vi "FlexRay_FR_Tab.vi"(7 "Fold Data":bool, 8 "error in (no error)":errorcluster, 9 "FR_Buffer":T1[](array[typedef]), 10 "FlexRay_Data IN":T2={"Communication message"={"Sender"="", "receiver"="", "message"="", "data"=variant}, "error in"={"status"=FALSE, "code"=0, "source"=""}, "Data"={"FR_Frame_Buffer"=[], "Config"={"DLL_PATH"=path "", "Project_PATH"=path "", "BLF_Log_PATH"=path "", "Read message type"=1, "Channel"=0, "REC_Channel"=0, "ChannelMask"=0, "ActualPayloadLength"=0, "CycleNumber"=0, "SlotId"=0, "Send_Array"=[1, 2, 3, 4, 5, 6, 7, 8, 9, 10, 11]}, "AsynCall?"=FALSE, "XML_Data"={"XML Path"=path "", "XML loading channel"=0}, "DataBase_array"=refnum}} {"Data"."XML_Data"."XML loading channel" items=["CHN1", "CHN2", "CHN3", "CHN4", "CHN5", "CHN6", "CHN7", "CHN8", "CHN9", "CHN10", "CHN11", "CHN12", "CHN13", "CHN14", "CHN15", "CHN16", "CHN17", "CHN18", "CHN19", "CHN20", "CHN21", "CHN22", "CHN23", "CHN24", "CHN25", "CHN26", "CHN27", "CHN28", "CHN29", "CHN30", "CHN31", "CHN32"]; "Data"."Config"."Send_Array" format="%.0x"; "Data"."Config"."ChannelMask" items=["reserved", "A", "B", "AB"]; "Data"."Config"."REC_Channel" items=["CHN1", "CHN2", "CHN3", "CHN4", "CHN5", "CHN6", "CHN7", "CHN8", "CHN9", "CHN10", "CHN11", "CHN12", "CHN13", "CHN14", "CHN15", "CHN16", "CHN17", "CHN18", "CHN19", "CHN20", "CHN21", "CHN22", "CHN23", "CHN24", "CHN25", "CHN26", "CHN27", "CHN28", "CHN29", "CHN30", "CHN31", "CHN32"]; "Data"."Config"."Channel" items=["CHN1", "CHN2", "CHN3", "CHN4", "CHN5", "CHN6", "CHN7", "CHN8", "CHN9", "CHN10", "CHN11", "CHN12", "CHN13", "CHN14", "CHN15", "CHN16", "CHN17", "CHN18", "CHN19", "CHN20", "CHN21", "CHN22", "CHN23", "CHN24", "CHN25", "CHN26", "CHN27", "CHN28", "CHN29", "CHN30", "CHN31", "CHN32"]; "Data"."Config"."Read message type" items=["Only read received messages", "Receive&send messages"]}, 11 "MulticolumnListbox in":refnum<vi>) -> (2 "FlexRay_Data":T2={"Communication message"={"Sender"="", "receiver"="", "message"="", "data"=variant}, "error in"={"status"=FALSE, "code"=0, "source"=""}, "Data"={"FR_Frame_Buffer"=[], "Config"={"DLL_PATH"=path "", "Project_PATH"=path "", "BLF_Log_PATH"=path "", "Read message type"=1, "Channel"=0, "REC_Channel"=0, "ChannelMask"=0, "ActualPayloadLength"=0, "CycleNumber"=0, "SlotId"=0, "Send_Array"=[1, 2, 3, 4, 5, 6, 7, 8, 9, 10, 11]}, "AsynCall?"=FALSE, "XML_Data"={"XML Path"=path "", "XML loading channel"=0}, "DataBase_array"=refnum}} {"Data"."XML_Data"."XML loading channel" items=["CHN1", "CHN2", "CHN3", "CHN4", "CHN5", "CHN6", "CHN7", "CHN8", "CHN9", "CHN10", "CHN11", "CHN12", "CHN13", "CHN14", "CHN15", "CHN16", "CHN17", "CHN18", "CHN19", "CHN20", "CHN21", "CHN22", "CHN23", "CHN24", "CHN25", "CHN26", "CHN27", "CHN28", "CHN29", "CHN30", "CHN31", "CHN32"]; "Data"."Config"."Send_Array" format="%.0x"; "Data"."Config"."ChannelMask" items=["reserved", "A", "B", "AB"]; "Data"."Config"."REC_Channel" items=["CHN1", "CHN2", "CHN3", "CHN4", "CHN5", "CHN6", "CHN7", "CHN8", "CHN9", "CHN10", "CHN11", "CHN12", "CHN13", "CHN14", "CHN15", "CHN16", "CHN17", "CHN18", "CHN19", "CHN20", "CHN21", "CHN22", "CHN23", "CHN24", "CHN25", "CHN26", "CHN27", "CHN28", "CHN29", "CHN30", "CHN31", "CHN32"]; "Data"."Config"."Channel" items=["CHN1", "CHN2", "CHN3", "CHN4", "CHN5", "CHN6", "CHN7", "CHN8", "CHN9", "CHN10", "CHN11", "CHN12", "CHN13", "CHN14", "CHN15", "CHN16", "CHN17", "CHN18", "CHN19", "CHN20", "CHN21", "CHN22", "CHN23", "CHN24", "CHN25", "CHN26", "CHN27", "CHN28", "CHN29", "CHN30", "CHN31", "CHN32"]; "Data"."Config"."Read message type" items=["Only read received messages", "Receive&send messages"]})   [LabVIEW 2014]
uses:
  Typedef/TLibFLexRay.ctl
  Typedef/FlexRay_Data.ctl
  Typedef/FlexRay_Config.ctl
  DataBase/Typedef/CAN/TCANSignal.ctl
  DataBase/Typedef/LIN/TLINSignal.ctl
  DataBase/Typedef/FlexRay/TFlexRaySignal.ctl
  DataBase/Typedef/TDBSignalProperties.ctl
  DataBase/Typedef/TDBFrameProperties.ctl
  DataBase/Typedef/TDBECUProperties.ctl
  DataBase/Typedef/TDBProperties.ctl
  DataBase/Typedef/DataBase_array.ctl
  DataBase/Typedef/DataBase_array_index.ctl
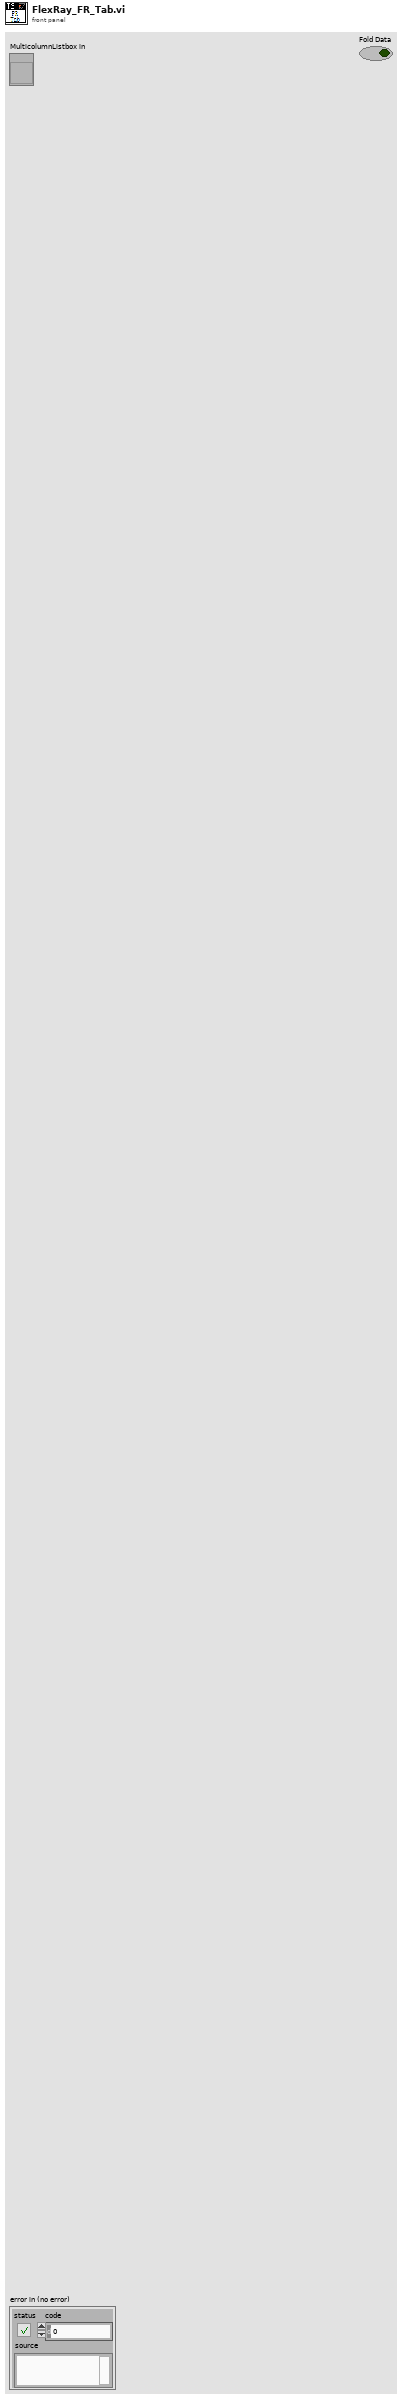
[diagram p1: front panel]
types:
  T1 = typedef "TLibFLexRay.ctl" = cluster{"FIdxChn":u8, "FChannelMask":u8, "FDir":u8, "FPayloadLength":u8, "FActualPayloadLength":u8, "FCycleNumber":u8, "FCCType":u8, "FFrameType":u8, "FHeaderCRCA":u16, "FHeaderCRCB":u16, "FFrameStateInfo":u16, "FSlotId":u16, "FFrameFlags":u32, "FFrameCRC":u32, "FReserved1":u64, "FReserved2":u64, "FTimeUs":u64, "FData":cluster{"数值":u8, "数值 9":u8, "数值 17":u8, "数值 25":u8, "数值 33":u8, "数值 41":u8, "数值 49":u8, "数值 57":u8, "数值 65":u8, "数值 73":u8, "数值 81":u8, "数值 89":u8, "数值 97":u8, "数值 105":u8, "数值 98":u8, "数值 99":u8, "数值 2":u8, "数值 10":u8, "数值 18":u8, "数值 26":u8, "数值 34":u8, "数值 42":u8, "数值 50":u8, "数值 58":u8, "数值 66":u8, "数值 74":u8, "数值 82":u8, "数值 90":u8, "数值 100":u8, "数值 106":u8, "数值 101":u8, "数值 102":u8, "数值 3":u8, "数值 11":u8, "数值 19":u8, "数值 27":u8, "数值 35":u8, "数值 43":u8, "数值 51":u8, "数值 59":u8, "数值 67":u8, "数值 75":u8, "数值 83":u8, "数值 91":u8, "数值 103":u8, "数值 107":u8, "数值 104":u8, "数值 108":u8, "数值 4":u8, "数值 12":u8, "数值 20":u8, "数值 28":u8, "数值 36":u8, "数值 44":u8, "数值 52":u8, "数值 60":u8, "数值 68":u8, "数值 76":u8, "数值 84":u8, "数值 92":u8, "数值 109":u8, "数值 110":u8, "数值 111":u8, "数值 112":u8, "数值 5":u8, "数值 13":u8, "数值 21":u8, "数值 29":u8, "数值 37":u8, "数值 45":u8, "数值 53":u8, "数值 61":u8, "数值 69":u8, "数值 77":u8, "数值 85":u8, "数值 93":u8, "数值 113":u8, "数值 114":u8, "数值 115":u8, "数值 116":u8, "数值 6":u8, "数值 14":u8, "数值 22":u8, "数值 30":u8, "数值 38":u8, "数值 46":u8, "数值 54":u8, "数值 62":u8, "数值 70":u8, "数值 78":u8, "数值 86":u8, "数值 94":u8, "数值 117":u8, "数值 118":u8, "数值 119":u8, "数值 120":u8, "数值 7":u8, "数值 15":u8, "数值 23":u8, "数值 31":u8, "数值 39":u8, "数值 47":u8, "数值 55":u8, "数值 63":u8, "数值 71":u8, "数值 79":u8, "数值 87":u8, "数值 95":u8, "数值 121":u8, "数值 122":u8, "数值 123":u8, "数值 124":u8, "数值 8":u8, "数值 16":u8, "数值 24":u8, "数值 32":u8, "数值 40":u8, "数值 48":u8, "数值 56":u8, "数值 64":u8, "数值 72":u8, "数值 80":u8, "数值 88":u8, "数值 96":u8, "数值 125":u8, "数值 126":u8, "数值 127":u8, "数值 128":u8, "数值 129":u8, "数值 130":u8, "数值 131":u8, "数值 132":u8, "数值 133":u8, "数值 134":u8, "数值 135":u8, "数值 136":u8, "数值 137":u8, "数值 138":u8, "数值 139":u8, "数值 140":u8, "数值 141":u8, "数值 142":u8, "数值 143":u8, "数值 144":u8, "数值 145":u8, "数值 146":u8, "数值 147":u8, "数值 148":u8, "数值 149":u8, "数值 150":u8, "数值 151":u8, "数值 152":u8, "数值 153":u8, "数值 154":u8, "数值 155":u8, "数值 156":u8, "数值 157":u8, "数值 158":u8, "数值 159":u8, "数值 160":u8, "数值 161":u8, "数值 162":u8, "数值 163":u8, "数值 164":u8, "数值 165":u8, "数值 166":u8, "数值 167":u8, "数值 168":u8, "数值 169":u8, "数值 170":u8, "数值 171":u8, "数值 172":u8, "数值 173":u8, "数值 174":u8, "数值 175":u8, "数值 176":u8, "数值 177":u8, "数值 178":u8, "数值 179":u8, "数值 180":u8, "数值 181":u8, "数值 182":u8, "数值 183":u8, "数值 184":u8, "数值 185":u8, "数值 186":u8, "数值 187":u8, "数值 188":u8, "数值 189":u8, "数值 190":u8, "数值 191":u8, "数值 192":u8, "数值 193":u8, "数值 194":u8, "数值 195":u8, "数值 196":u8, "数值 197":u8, "数值 198":u8, "数值 199":u8, "数值 200":u8, "数值 201":u8, "数值 202":u8, "数值 203":u8, "数值 204":u8, "数值 205":u8, "数值 206":u8, "数值 207":u8, "数值 208":u8, "数值 209":u8, "数值 210":u8, "数值 211":u8, "数值 212":u8, "数值 213":u8, "数值 214":u8, "数值 215":u8, "数值 216":u8, "数值 217":u8, "数值 218":u8, "数值 219":u8, "数值 220":u8, "数值 221":u8, "数值 222":u8, "数值 223":u8, "数值 224":u8, "数值 225":u8, "数值 226":u8, "数值 227":u8, "数值 228":u8, "数值 229":u8, "数值 230":u8, "数值 231":u8, "数值 232":u8, "数值 233":u8, "数值 234":u8, "数值 235":u8, "数值 236":u8, "数值 237":u8, "数值 238":u8, "数值 239":u8, "数值 241":u8, "数值 242":u8, "数值 243":u8, "数值 244":u8, "数值 245":u8, "数值 246":u8, "数值 247":u8, "数值 248":u8, "数值 249":u8, "数值 250":u8, "数值 251":u8, "数值 252":u8, "数值 253":u8, "数值 254":u8, "数值 255":u8}}
  T2 = typedef "FlexRay_Data.ctl" = cluster{"Communication message":cluster{"Sender":string, "receiver":string, "message":string, "data":variant}, "error in":errorcluster, "Data":cluster{"FR_Frame_Buffer":T1[], "Config":T3, "AsynCall?":bool, "XML_Data":cluster{"XML Path":path, "XML loading channel":i32}, "DataBase_array":T4}}
  T3 = typedef "FlexRay_Config.ctl" = cluster{"DLL_PATH":path, "Project_PATH":path, "BLF_Log_PATH":path, "Read message type":u16, "Channel":i32, "REC_Channel":i32, "ChannelMask":u16, "ActualPayloadLength":u8, "CycleNumber":u8, "SlotId":u16, "Send_Array":u8[]}
  T4 = typedef "DataBase_array_index.ctl" = refnum<vi>
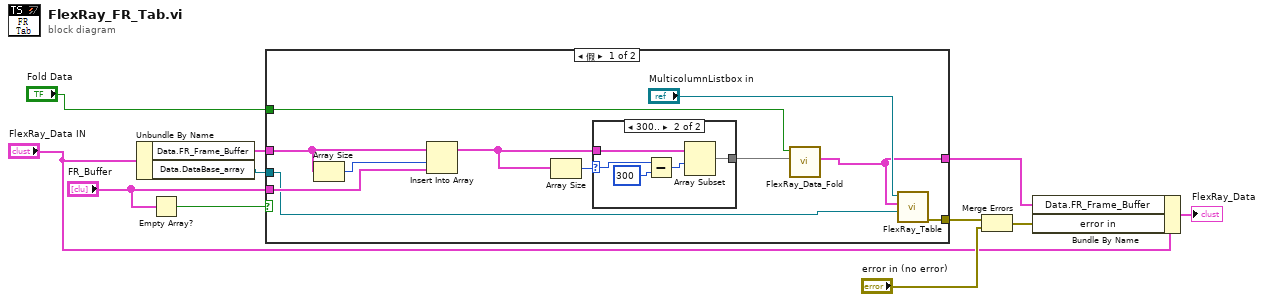
[diagram p0: block diagram]
diagram:
  n1 = Unbundle By Name("FlexRay_Data IN") -> ("Data.FR_Frame_Buffer"=w11:T1[], "Data.DataBase_array"=w1:T4)
  n2 = Empty Array?(array="FR_Buffer") -> (empty?=w9:bool)
  n3 = case shown="假" w9 {
    tunnel: [w15 w29] -> w8
    tunnel: w11 -> [w22 w29]
    tunnel: "FR_Buffer" -> [w17 _]
    tunnel: [w18 _] -> w6
    tunnel: "Fold Data" -> [w14 _]
    tunnel: w1 -> [w12 _]
    frame False {
      n4 = Array Size(array=w22) -> (size(s)=w20:i32)
      n5 = Insert Into Array(array=w22, index=w20, new element=w17) -> (w16:T1[])
      n6 = Array Size(array=w16) -> (size(s)=w21:i32)
      n7 = case shown="300.." w21 {
        selector: w21 -> [_ w28]
        tunnel: [w23 w26] -> w13
        tunnel: w16 -> [w23 w24]
        frame 0, Default {
        }
        frame 300.. {
          n8 = Subtract(x=w28, y=300) -> (x-y=w25:i32)
          n9 = Array Subset(array=w24, index=w25) -> (w26:T1[])  [unwired: 1 in]
        }
      }
      n10 = call "FlexRay_Data_Fold.vi"("FR_Buffer"=w13, "Fold Data"=w14) -> ("FR_Buffer out"=w15:T1[])  [unwired: 9 in]
      n11 = call "FlexRay_Table.vi"("DataBase_array"=w12, "FR_Buffer"=w15, "FlexRay_Data Ref"="MulticolumnListbox in") -> ("错误输出"=w18:errorcluster)  [unwired: 8 in]
    }
    frame True {
    }
  }
  n12 = Merge Errors(w6, "error in (no error)") -> (w7:errorcluster)
  n13 = Bundle By Name(cluster="FlexRay_Data IN", "Data.FR_Frame_Buffer"=w8, "error in"=w7) -> (→"FlexRay_Data":T2)
